vi "Attack.vi"(8 "error in (no error)":errorcluster, 9 "Attack?":T2, 10 "Maze (0: Empty, -1: Enemy. >0: Teammate":i32[](array[numeric]), 11 "Mother in":refnum<class "Mother.lvclass">) -> (0 "error out":errorcluster, 1 "Direction":T1, 2 "Action":T3, 3 "Mother out":refnum<class "Mother.lvclass">, 4 "Enemy Found?":bool, 6 "Enemy Direction":T1)   [LabVIEW 2014, in "Mother.lvclass"]
uses:
  Mother.lvclass
  Direction Enum.ctl
  Action Enum.ctl
  Attack Options.ctl
  SquareBattle.lvclass
panel:
  in  "Status":string
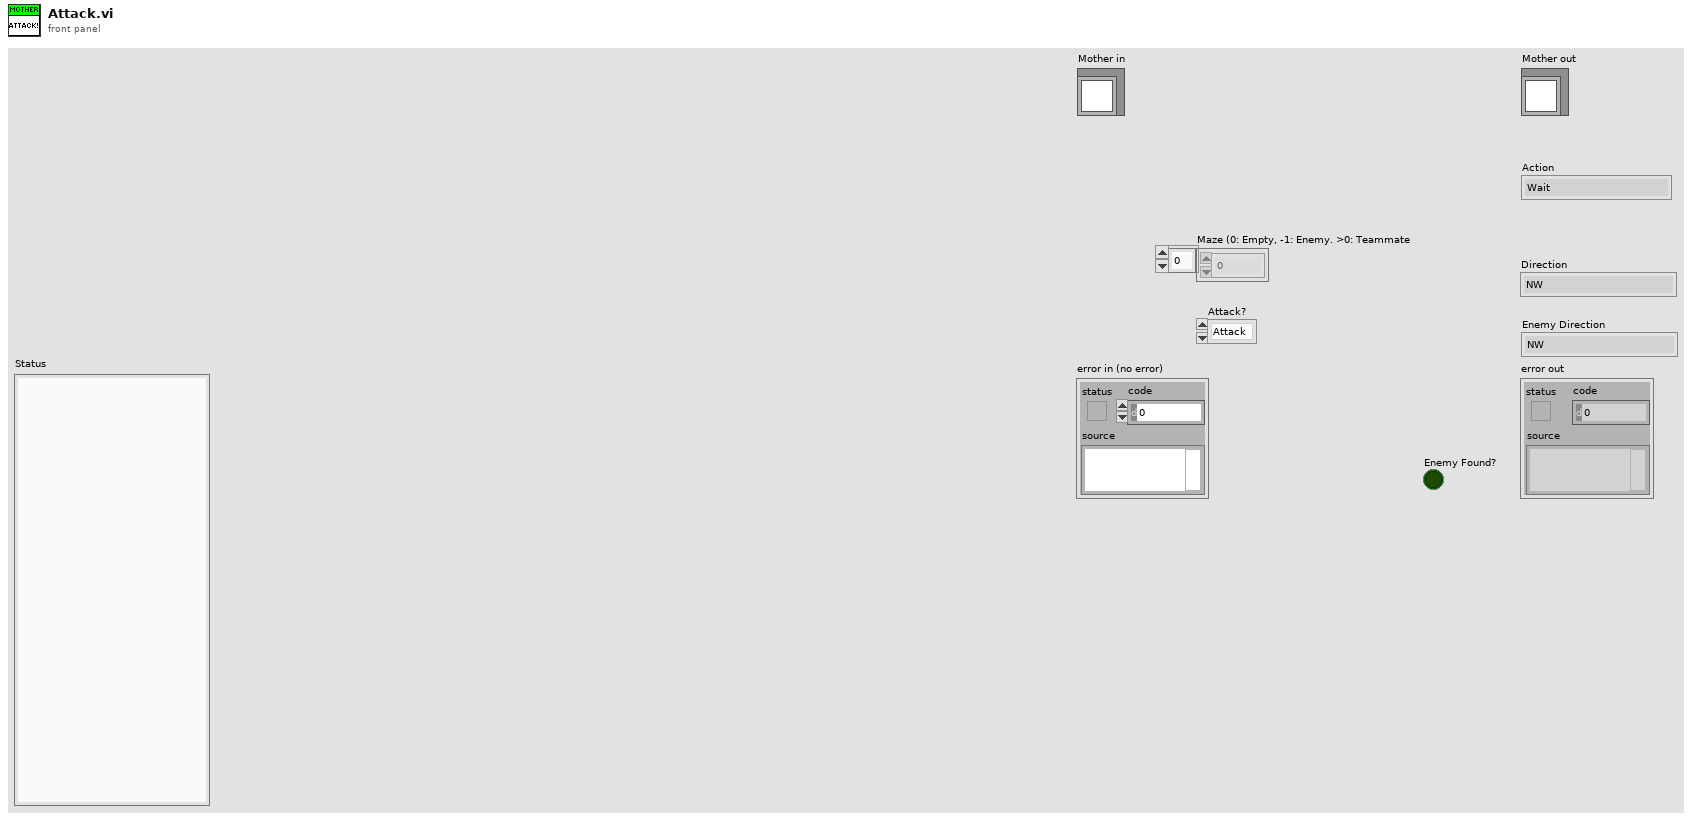
[diagram p1: front panel]
types:
  T1 = typedef "SquareBattle.lvclass/Direction Enum.ctl" = enum16{"NW", "N", "NE", "E", "SE", "S", "SW", "W"}
  T2 = typedef "Mother.lvclass/Attack Options.ctl" = enum16{"Attack", "Run", "Distract"}
  T3 = typedef "SquareBattle.lvclass/Action Enum.ctl" = enum16{"Wait", "Move", "Attack", "Replicate"}
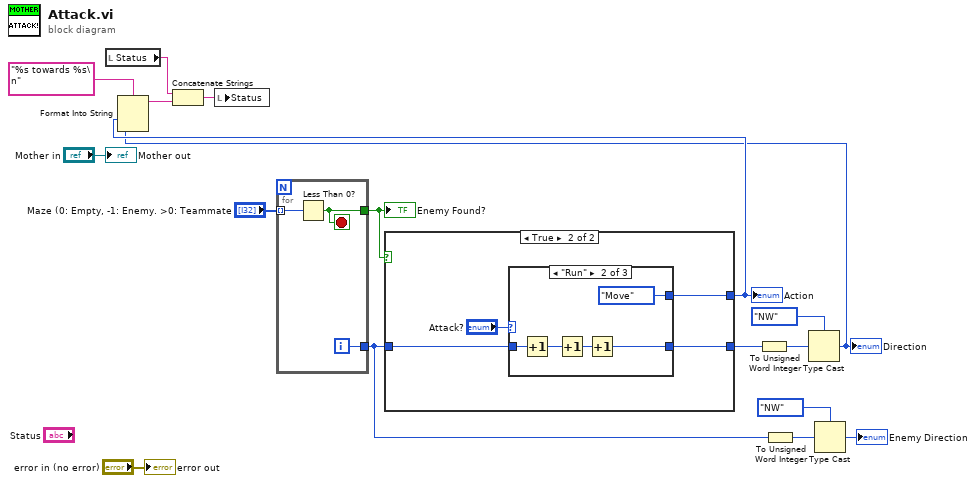
[diagram p0: block diagram]
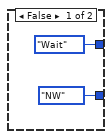
[diagram p2: hidden frame]
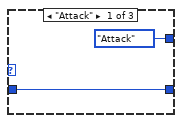
[diagram p3: hidden frame]
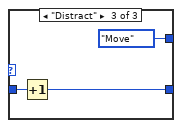
[diagram p4: hidden frame]
diagram:
  n1 = local read "Status"() -> (w10:string)
  n2 = for {
    tunnel: "Maze (0: Empty, -1: Enemy. >0: Teammate" -> [w19] mode=indexing
    tunnel: [w18] -> w1
    tunnel: [w20] -> w15
    i -> [w18]
    stop <- w20 stop-if-true
    n3 = Less Than 0?(x=w19) -> (x < 0?=w20:bool)
  }
  "Enemy Found?" <- w15
  n4 = case shown="True" w15 {
    tunnel: [Action_Enum."Wait" ("Action") w26] -> w6
    tunnel: [Direction_Enum."NW" ("Direction") w24] -> w13
    tunnel: w1 -> [_ w23]
    frame False {
    }
    frame True {
      n5 = case shown="\"Run\"" "Attack?" {
        tunnel: [Action_Enum."Attack" ("Action") Action_Enum."Move" ("Action") Action_Enum."Move" ("Action")] -> w26
        tunnel: [w27 w29 w34] -> w24
        tunnel: w23 -> [w27 w32 w35]
        frame "Attack" {
        }
        frame "Run" {
          n6 = Increment(x=w32) -> (x+1=w31:i32)
          n7 = Increment(x=w31) -> (x+1=w30:i32)
          n8 = Increment(x=w30) -> (x+1=w29:i32)
        }
        frame "Distract" {
          n9 = Increment(x=w35) -> (x+1=w34:i32)
        }
      }
    }
  }
  "Action" <- w6
  n10 = To Unsigned Word Integer(number=w13) -> (unsigned 16bit integer=w12:u16)
  n11 = To Unsigned Word Integer(number=w1) -> (unsigned 16bit integer=w2:u16)
  n12 = Type Cast(type=Direction_Enum."NW" ("Direction"), x=w12) -> (*(type *) &x=w5:T1)
  "Direction" <- w5
  n13 = Format Into String(format string="%s towards %s\n", w6, w5) -> (resulting string=w7:string)  [unwired: 2 in, 1 out]
  n14 = Concatenate Strings(w10, w7) -> (w9:string)
  n15 = local write "Status"(w9) -> ()
  n16 = Type Cast(type=Direction_Enum."NW" ("Direction"), x=w2) -> (*(type *) &x=→"Enemy Direction":T1)
  "error out" <- "error in (no error)"
  "Mother out" <- "Mother in"
